vi "PCO_RecorderSetAutoExposure.vi"(0 "phRec":u64, 1 "dwMinExposure":u32=500, 2 "wExpBase":u16(ring)=1 items=["ns", "us", "ms"], 5 "phCam":u64, 7 "bAutoExpState":bool, 9 "wSmoothness":u16=1, 11 "error in (no error)":errorcluster {"code" format="%x"}, 12 "dwMaxExposure":u32=100000) -> (4 "phRec out":u64, 6 "ErrorMessage":i32 format="%x", 15 "error out":errorcluster {"code" format="%x"})   [LabVIEW 2019, in "Recorder.lvlib"]
doc: "int WINAPI PCO_RecorderSetAutoExposure(HANDLE phRec, HANDLE phCam, bool autoExpState, WORD smoothness, DWORD minExposure, DWORD maxExposure, WORD expBase);"
uses:
  Recorder.lvlib
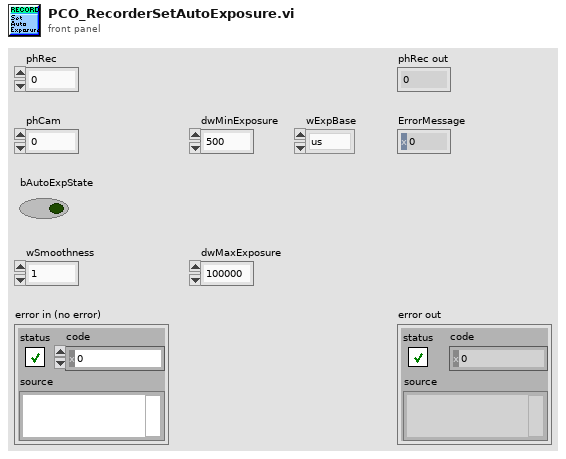
[diagram p1: front panel]
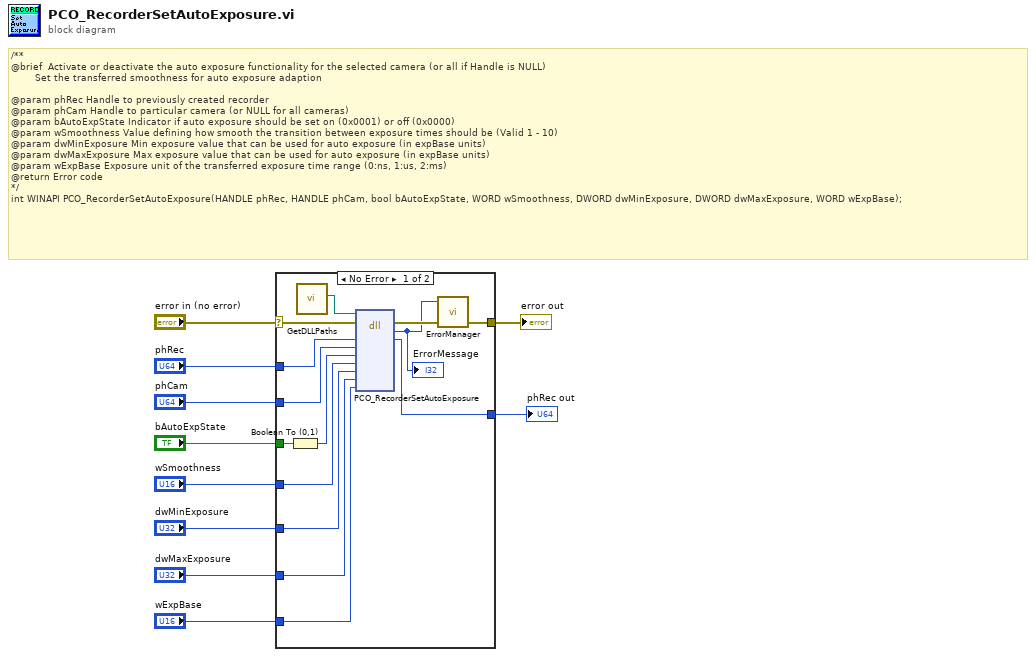
[diagram p0: block diagram]
diagram:
  # "/**\n@brief \tActivate or deactivate the auto exposure functionality for the selected camera (or all if Handle is NULL)\n        Set the transferred smoothness for auto exposure adaption\n\n@param phRec Handle to previously created recorder\n@param phCam Handle to particular camera (or NULL for all cameras)\n@param bAutoExpState Indicator if auto exposure should be set on (0x0001) or off (0x0000)\n@param wSmoothness Value defining how smooth the transition between exposure times should be (Valid 1 - 10)\n@param dwMinExposure Min exposure value that can be used for auto exposure (in expBase units)\n@param dwMaxExposure Max exposure value that can be used for auto exposure (in expBase units)\n@param wExpBase Exposure unit of the transferred exposure time range (0:ns, 1:us, 2:ms)\n@return Error code\n*/\nint WINAPI PCO_RecorderSetAutoExposure(HANDLE phRec, HANDLE phCam, bool bAutoExpState, WORD wSmoothness, DWORD dwMinExposure, DWORD dwMaxExposure, WORD wExpBase);"
  n1 = case shown="No Error" "error in (no error)" {
    selector: "error in (no error)" -> [w15 w26]
    tunnel: "phRec" -> [w24 w25]
    tunnel: [w23 w25] -> w9
    tunnel: "phCam" -> [w22 _]
    tunnel: "bAutoExpState" -> [w21 _]
    tunnel: "wSmoothness" -> [w19 _]
    tunnel: "dwMinExposure" -> [w18 _]
    tunnel: "dwMaxExposure" -> [w17 _]
    tunnel: "wExpBase" -> [w16 _]
    tunnel: [w13 w26] -> w2
    frame No Error {
      n2 = Boolean To (0,1)(Boolean=w21) -> (0, 1=w20:i16)
      n3 = call "GetDLLPaths.vi"() -> ("PCO_Recorder_Path"=w11:path)  [unwired: 8 in, 3 out]
      n4 = dll-call lib="?" fn="PCO_RecorderSetAutoExposure"(path in=w11, error in=w15, "phRec"=w24, "phCam"=w22, "bAutoExpState"=w20, "wSmoothness"=w19, "dwMinExposure"=w18, "dwMaxExposure"=w17, "wExpBase"=w16) -> (error out=w14:errorcluster, "return type"=w12:i32, "phRec"=w23:u64)  [unwired: 7 in, 1 out]
      "ErrorMessage" <- w12
      n5 = call "ErrorManager.vi"("error in (no error)"=w14, "error code"=w12) -> ("error out"=w13:errorcluster)  [unwired: 2 in, 1 out]
    }
    frame Error {
    }
  }
  "phRec out" <- w9
  "error out" <- w2
